vi "GetTerms3.vi"(0 "XRef":T10, 1 "State In":T9) -> (14 "Terms":T8)   [LabVIEW 2010, in "CData Flatten XNode.xnode"]
doc: "This ability VI is used to describe your terminals to LabVIEW. Terms is an array of clusters describing the XNode's terminals.\n ID: A unique string identifying the terminal.\n Name: The name of the terminal visible to the user. Remember to localize it.\n Type: The data type of the terminal (as a Variant). The data put in the variant will be used as the default for the input terminal if it's left unwired.\n Bounds: A rectangle defining the bounds of the terminal relative to the bounds of the XNode. The bounds must be within the bounds of the XNode, and for whiskers to draw properly, they must be flush with at least one side of the XNode.\n Input?: Indicates whether or not this terminals is an input.\n Required?: Indicates whether the user must wire this terminal for the XNode to not be broken. Ignored on outputs.\n Recommended?: Indicates whether the terminal is recommended.\n Hidden?: Indicates whether the terminal is hidden. When a terminal is hidden, it cannot be wired to via user interaction or scripting. However, if it is already wired to when the hidden flag is changed to true, it will remain wired.\n Adaptive?: Indicates that the term should change to match the type of its source if it is wired.\n Direction?: Indicates what direction the wire stub should point. Choose auto to let LV decide based on the terms bounds being on the nodes edge.\n \n The IDs are used by LabVIEW to keep track of your terminals. When you respecify your terminals, LabVIEW can tell whther terminals are new, deleted, or moved by the unique IDs. The order is irrelevant. If you move a terminal, then any wire connected to it will move with it.\n \n If you want to update your terminals, you should return the UpdateTerms reply in one of your ability VIs.\n\nDefault behavior: None.\n\nThis ability does not provide UI and OS messages are not handled."
uses:
  CData Flatten XNode.xnode
  <vilib>/XNodeSupport/XNodeXNodeRef.ctl
  State.ctl
  <vilib>/XNodeSupport/XNodeTerm3Array.ctl
  <vilib>/XNodeSupport/XNodeTerm3.ctl
  <vilib>/XNodeSupport/XNodeString.ctl
  <vilib>/XNodeSupport/XNodeVariant.ctl
  <vilib>/XNodeSupport/XNodeRect32.ctl
  <vilib>/XNodeSupport/XNodeInt.ctl
  <vilib>/XNodeSupport/XNodeBool.ctl
  <vilib>/XNodeSupport/XNodeTermDirection.ctl
  <vilib>/XNodeSupport/NI_XNodeSupport.lvlib
panel:
  in  "Array":T1[](array[typedef])=[{"Name"="error out", "Id"="error out", "Type"=variant(errorcluster {"status"=FALSE, "code"=0, "source"=""}), "Bounds"={"Left"=24, "Top"=24, "Right"=32, "Bottom"=32}, "Input?"=FALSE, "Required?"=FALSE, "Recommended?"=FALSE, "Adaptive?"=FALSE, "Hidden?"=FALSE, "Direction"=enum."Auto", "Break Wire?"=FALSE}, {"Name"="value", "Id"="value", "Type"=variant(cluster{} {}), "Bounds"={"Left"=24, "Top"=16, "Right"=32, "Bottom"=24}, "Input?"=FALSE, "Required?"=FALSE, "Recommended?"=FALSE, "Adaptive?"=TRUE, "Hidden?"=FALSE, "Direction"=enum."Auto", "Break Wire?"=FALSE}, {"Name"="rest of the binary string", "Id"="rest of the binary string", "Type"=variant(string ""), "Bounds"={"Left"=24, "Top"=8, "Right"=32, "Bottom"=16}, "Input?"=FALSE, "Required?"=FALSE, "Recommended?"=FALSE, "Adaptive?"=FALSE, "Hidden?"=FALSE, "Direction"=enum."Auto", "Break Wire?"=FALSE}, {"Name"="type", "Id"="type", "Type"=variant(cluster{} {}), "Bounds"={"Left"=8, "Top"=0, "Right"=16, "Bottom"=16}, "Input?"=TRUE, "Required?"=FALSE, "Recommended?"=FALSE, "Adaptive?"=TRUE, "Hidden?"=FALSE, "Direction"=enum."Auto", "Break Wire?"=FALSE}, {"Name"="error in (no error)", "Id"="error in (no error)", "Type"=variant(errorcluster {"status"=FALSE, "code"=0, "source"=""}), "Bounds"={"Left"=0, "Top"=24, "Right"=8, "Bottom"=32}, "Input?"=TRUE, "Required?"=FALSE, "Recommended?"=FALSE, "Adaptive?"=FALSE, "Hidden?"=FALSE, "Direction"=enum."Auto", "Break Wire?"=FALSE}, {"Name"="binary string", "Id"="binary string", "Type"=variant(string ""), "Bounds"={"Left"=0, "Top"=8, "Right"=8, "Bottom"=16}, "Input?"=TRUE, "Required?"=FALSE, "Recommended?"=FALSE, "Adaptive?"=FALSE, "Hidden?"=FALSE, "Direction"=enum."Auto", "Break Wire?"=FALSE}]
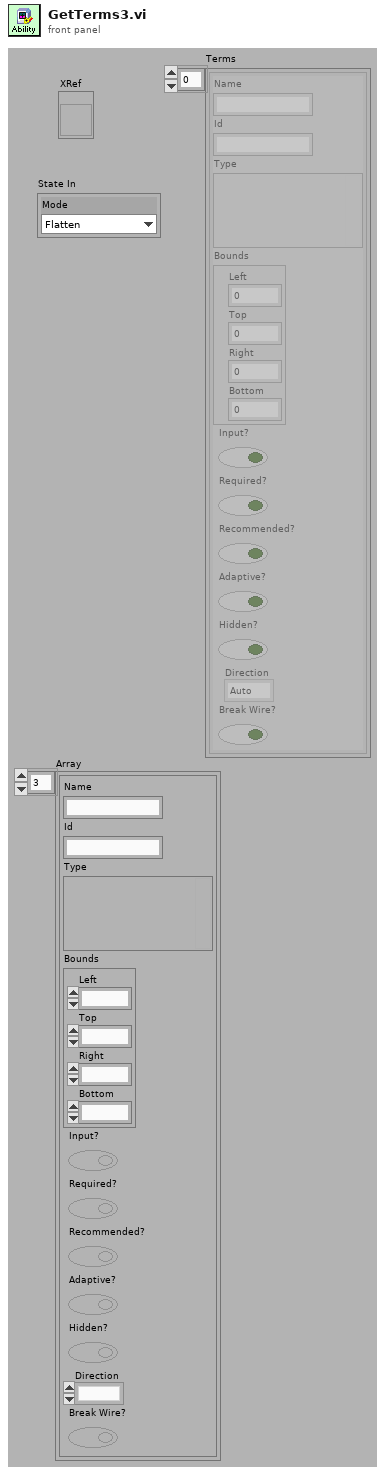
[diagram p1: front panel]
types:
  T1 = typedef "NI_XNodeSupport.lvlib/XNodeTerm3.ctl" = cluster{"Name":T2, "Id":T2, "Type":T3, "Bounds":T4, "Input?":T6, "Required?":T6, "Recommended?":T6, "Adaptive?":T6, "Hidden?":T6, "Direction":T7, "Break Wire?":T6}
  T2 = typedef "NI_XNodeSupport.lvlib/XNodeString.ctl" = string
  T3 = typedef "NI_XNodeSupport.lvlib/XNodeVariant.ctl" = variant
  T4 = typedef "NI_XNodeSupport.lvlib/XNodeRect32.ctl" = cluster{"Left":T5, "Top":T5, "Right":T5, "Bottom":T5}
  T5 = typedef "NI_XNodeSupport.lvlib/XNodeInt.ctl" = i32
  T6 = typedef "NI_XNodeSupport.lvlib/XNodeBool.ctl" = bool
  T7 = typedef "NI_XNodeSupport.lvlib/XNodeTermDirection.ctl" = enum32{"Auto", "Up", "Down", "Left", "Right", "Center"}
  T8 = typedef "NI_XNodeSupport.lvlib/XNodeTerm3Array.ctl" = T1[]
  T9 = typedef "CData Flatten XNode.xnode/State.ctl" = cluster{"Mode":enum16{"Flatten", "Unflatten"}}
  T10 = typedef "NI_XNodeSupport.lvlib/XNodeXNodeRef.ctl" = refnum<vi>
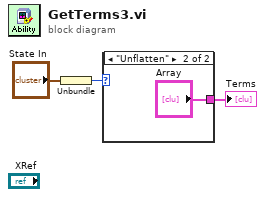
[diagram p0: block diagram]
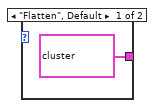
[diagram p2: hidden frame]
diagram:
  n1 = Unbundle("State In") -> ("Mode"=w2:enum16{"Flatten", "Unflatten"})
  n2 = case shown="\"Unflatten\"" w2 {
    tunnel: [T1[] [{"Name"="error out", "Id"="error out", "Type"=variant(errorcluster {"status"=FALSE, "code"=0, "source"=""}), "Bounds"={"Left"=24, "Top"=24, "Right"=32, "Bottom"=32}, "Input?"=FALSE, "Required?"=FALSE, "Recommended?"=FALSE, "Adaptive?"=FALSE, "Hidden?"=FALSE, "Direction"=enum."Auto", "Break Wire?"=FALSE}, {"Name"="data string", "Id"="data string", "Type"=variant(string ""), "Bounds"={"Left"=24, "Top"=8, "Right"=32, "Bottom"=16}, "Input?"=FALSE, "Required?"=FALSE, "Recommended?"=FALSE, "Adaptive?"=FALSE, "Hidden?"=FALSE, "Direction"=enum."Auto", "Break Wire?"=FALSE}, {"Name"="error in (no error)", "Id"="error in (no error)", "Type"=variant(errorcluster {"status"=FALSE, "code"=0, "source"=""}), "Bounds"={"Left"=0, "Top"=24, "Right"=8, "Bottom"=32}, "Input?"=TRUE, "Required?"=FALSE, "Recommended?"=FALSE, "Adaptive?"=FALSE, "Hidden?"=FALSE, "Direction"=enum."Auto", "Break Wire?"=FALSE}, {"Name"="anything", "Id"="anything", "Type"=variant(cluster{} {}), "Bounds"={"Left"=0, "Top"=8, "Right"=8, "Bottom"=16}, "Input?"=TRUE, "Required?"=TRUE, "Recommended?"=FALSE, "Adaptive?"=TRUE, "Hidden?"=FALSE, "Direction"=enum."Auto", "Break Wire?"=FALSE}] ("Array") "Array"] -> w1
    frame "Flatten", Default {
    }
    frame "Unflatten" {
    }
  }
  "Terms" <- w1
